vi "vi.vi"(4 "timeout (s)":dbl=10.0 format="%0.2f", 5 "error in":errorcluster, 7 "stop (T)":bool=TRUE) -> (14 "task out":refnum<k21>, 15 "data":dynamicdata(waveform), 19 "error out":errorcluster)   [LabVIEW 2010]
doc: "Creates, edits, and runs tasks using NI-DAQmx. Refer to the NI-DAQmx Readme for a complete listing of devices NI-DAQmx supports.\n\nWhen you place this Express VI on the block diagram, the DAQ Assistant launches to create a new task. After you create a task, you can double-click the DAQ Assistant Express VI to edit that task. For continuous measurement or generation, place a while loop around the DAQ Assistant Express VI.\n\nFor continuous single-point input or output, the DAQ Assistant Express VI might not provide optimal performance. Refer to the Cont Acq&Graph Voltage-Single Point Optimization VI in examples\\DAQmx\\Analog In\\Measure Voltage.llb for an example of techniques to create higher-performance, single-point I/O applications."
uses:
  <vilib>/DAQmx/create/channels.llb/DAQmx Create Channel (TEDS-AI-Voltage-Basic).vi
  <vilib>/DAQmx/create/channels.llb/DAQmx Create Channel (AI-Voltage-Basic).vi
  <vilib>/DAQmx/read.llb/DAQmx Read.vi
  <vilib>/DAQmx/read.llb/DAQmx Read (Analog 1D DBL NChan 1Samp).vi
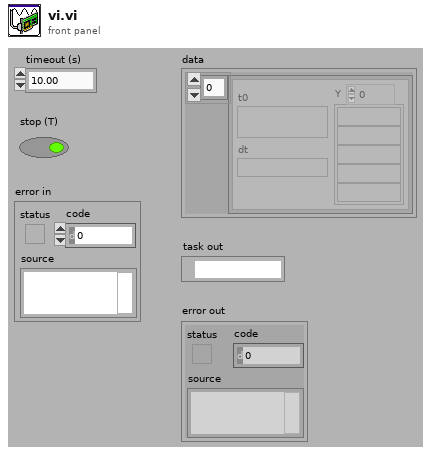
[diagram p1: front panel]
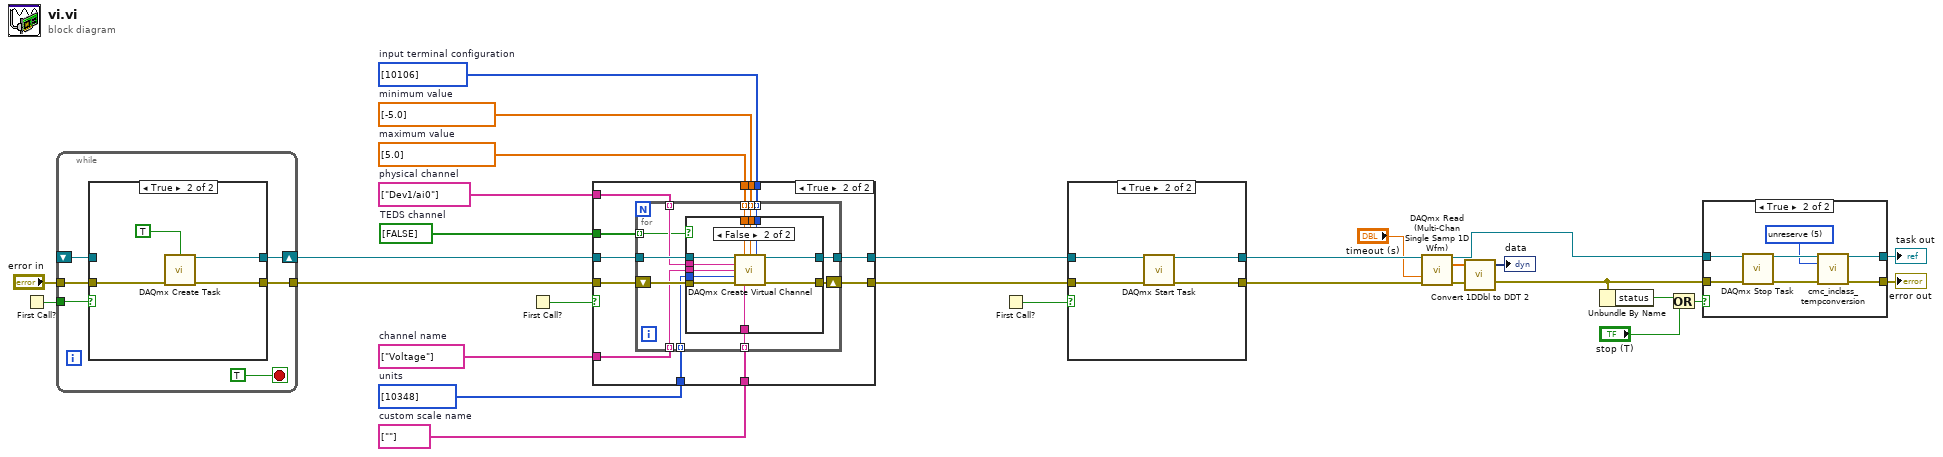
[diagram p0: block diagram]
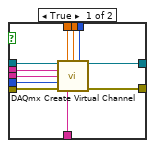
[diagram p5: hidden frame]
diagram:
  w15 = bool[] [FALSE]  # TEDS channel
  w16 = string[] [""]  # custom scale name
  w17 = i32[] [10348] items=["Volts"=10348, "From TEDS"=12516, "From Custom Scale"=10065]  # units
  w18 = string[] ["Voltage"]  # channel name
  w19 = string[] ["Dev1/ai0"]  # physical channel
  w20 = dbl[] [5.0]  # maximum value
  w21 = dbl[] [-5.0]  # minimum value
  w22 = i32[] [10106] items=["default"=-1, "RSE"=10083, "NRSE"=10078, "Differential"=10106, "Pseudodifferential"=12529]  # input terminal configuration
  n1 = First Call?() -> (First Call?: T/F=w28:bool)
  n2 = while {
    shift-right: [w33] -> w24
    shift-left: _ -> [w32]
    tunnel: w28 -> [w34]
    tunnel: [w31] -> w27
    tunnel: "error in" -> [w30]
    stop <- TRUE stop-if-true
    n3 = case shown="True" w34 {
      tunnel: [w36 w40] -> w33
      tunnel: w32 -> [w36 _]
      tunnel: [w35 w39] -> w31
      tunnel: w30 -> [w35 w37]
      frame False {
      }
      frame True {
        n4 = call <vilib>:"DAQmx Create Task.vi"("auto cleanup"=TRUE, "error in"=w37) -> ("task out"=w40:refnum<k21>, "error out"=w39:errorcluster)  [unwired: 12 in]
      }
    }
  }
  n5 = First Call?() -> (First Call?: T/F=w25:bool)
  n6 = case shown="True" w25 {
    tunnel: [w42 w52] -> w13
    tunnel: w24 -> [w42 w54]
    tunnel: [w41 w51] -> w23
    tunnel: w27 -> [w41 w53]
    tunnel: w22 -> [_ w50]
    tunnel: w21 -> [_ w49]
    tunnel: w20 -> [_ w48]
    tunnel: w19 -> [_ w47]
    tunnel: w18 -> [_ w46]
    tunnel: w17 -> [_ w45]
    tunnel: w16 -> [_ w44]
    tunnel: w15 -> [_ w43]
    frame False {
    }
    frame True {
      n7 = for {
        tunnel: w54 -> [w66]
        tunnel: [w64] -> w52
        tunnel: w50 -> [w62] mode=indexing
        tunnel: w49 -> [w61] mode=indexing
        tunnel: w48 -> [w60] mode=indexing
        tunnel: w47 -> [w59] mode=indexing
        tunnel: w46 -> [w58] mode=indexing
        tunnel: w45 -> [w57] mode=indexing
        tunnel: w44 -> [w56] mode=indexing
        shift-right: [w63] -> w51
        shift-left: w53 -> [w65]
        tunnel: w43 -> [w55] mode=indexing
        n8 = case shown="False" w55 {
          tunnel: w66 -> [w77 w88]
          tunnel: w65 -> [w76 w87]
          tunnel: [w75 w86] -> w64
          tunnel: [w74 w85] -> w63
          tunnel: w62 -> [w73 w84]
          tunnel: w61 -> [w72 w83]
          tunnel: w60 -> [w71 w82]
          tunnel: w59 -> [w70 w81]
          tunnel: w58 -> [w69 w80]
          tunnel: w57 -> [w68 w79]
          tunnel: w56 -> [w67 w78]
          frame True {
            n9 = call-poly <vilib>:"DAQmx Create Virtual Channel.vi"("task in"=w77, "maximum value"=w71, "minimum value"=w72, "input terminal configuration"=w73, "physical channels"=w70, "name to assign"=w69, "units"=w68, "error in"=w76, "custom scale name"=w67) -> ("task out"=w75:refnum<k21>, "error out"=w74:errorcluster)  [unwired: 5 in]
          }
          frame False {
            n10 = call-poly <vilib>:"DAQmx Create Virtual Channel.vi"("task in"=w88, "maximum value"=w82, "minimum value"=w83, "input terminal configuration"=w84, "physical channels"=w81, "name to assign"=w80, "units"=w79, "error in"=w87, "custom scale name"=w78) -> ("task out"=w86:refnum<k21>, "error out"=w85:errorcluster)  [unwired: 5 in]
          }
        }
      }
    }
  }
  n11 = First Call?() -> (First Call?: T/F=w14:bool)
  n12 = case shown="True" w14 {
    tunnel: [w90 w93] -> w10
    tunnel: w13 -> [w90 w94]
    tunnel: [w89 w91] -> w12
    tunnel: w23 -> [w89 w92]
    frame False {
    }
    frame True {
      n13 = call <vilib>:"DAQmx Start Task.vi"("task/channels in"=w94, "error in"=w92) -> ("task out"=w93:refnum<k21>, "error out"=w91:errorcluster)  [unwired: 12 in]
    }
  }
  n14 = call-poly "DAQmx Read (Multi-Chan Single Samp 1D Wfm).vi"("task/channels in"=w10, "timeout"="timeout (s)", "error in"=w12) -> ("task out"=w5:refnum<k21>, "data"=w8:dbl[], "error out"=w11:errorcluster)  [unwired: 10 in]
  n15 = call <vilib>:"Convert 1DDbl to DDT 2.vi"("Array"=w8) -> ("Dynamic Data Type"=→"data":dynamicdata)  [unwired: 3 in]
  n16 = Unbundle By Name(w11) -> ("status"=w3:bool)
  n17 = Or(x=w3, y="stop (T)") -> (x .or. y?=w1:bool)
  n18 = case shown="True" w1 {
    tunnel: [w96 w97] -> w6
    tunnel: w5 -> [w96 w103]
    tunnel: [w95 w100] -> w4
    tunnel: w11 -> [w95 w102]
    frame False {
    }
    frame True {
      w98 = 5 items=["verify"=2, "reserve"=4, "commit"=3, "unreserve"=5, "abort"=6] ("action")
      n19 = call <vilib>:"DAQmx Stop Task.vi"("task/channels in"=w103, "error in"=w102) -> ("task out"=w99:refnum<k21>, "error out"=w101:errorcluster)  [unwired: 12 in]
      n20 = call "cmc_inclass_tempconversion.vi"("task/channels in"=w99, "action"=w98, "error in"=w101) -> ("task out"=w97:refnum<k21>, "error out"=w100:errorcluster)  [unwired: 11 in]
    }
  }
  "task out" <- w6
  "error out" <- w4
